vi "Write Display Sec Listbox.vi"(8 "error in (no error)":errorcluster, 10 "Display Sec Listbox":refnum<vi>, 11 "TestSeqClass in":refnum<class "TestSeqClass.lvclass">) -> (0 "error out":errorcluster, 3 "TestSeqClass out":refnum<class "TestSeqClass.lvclass">)   [LabVIEW 2019]
uses:
  TestSeqClass.lvclass
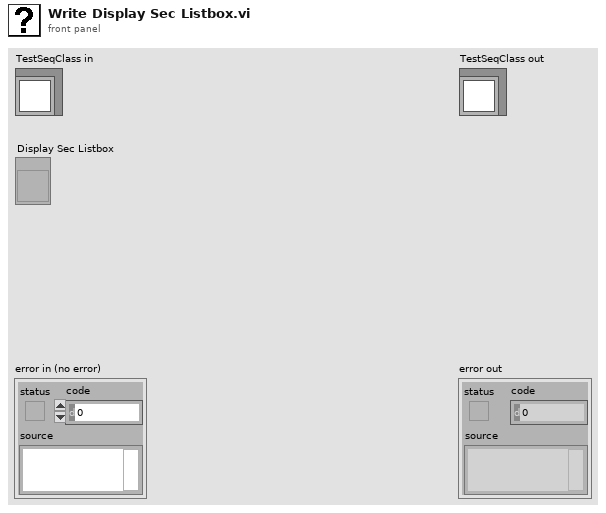
[diagram p1: front panel]
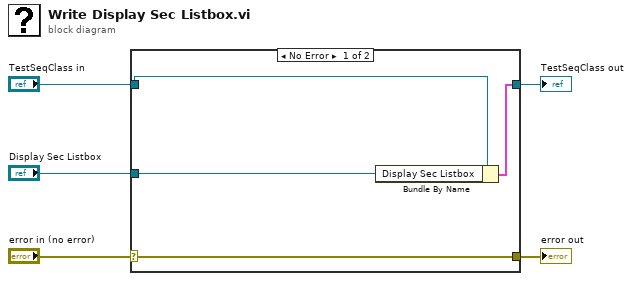
[diagram p0: block diagram]
diagram:
  n1 = case shown="No Error" "error in (no error)" {
    selector: "error in (no error)" -> [w9 w10]
    tunnel: [w9 w10] -> w4
    tunnel: [w7 w11] -> w2
    tunnel: "TestSeqClass in" -> [w8 w11]
    tunnel: "Display Sec Listbox" -> [w6 _]
    frame No Error {
      n2 = Bundle By Name(cluster=w8, "Display Sec Listbox"=w6) -> (w7:cluster{})
    }
    frame Error {
    }
  }
  "error out" <- w4
  "TestSeqClass out" <- w2
